vi "panelResize_tdms.vi"(4 "error in (no error)":errorcluster, 5 "NewBnds":T2, 7 "control refs":T1) -> (0 "error out":errorcluster)   [LabVIEW 2020]
uses:
  <vilib>/Utility/miscctls.llb/LVRectTypeDef.ctl
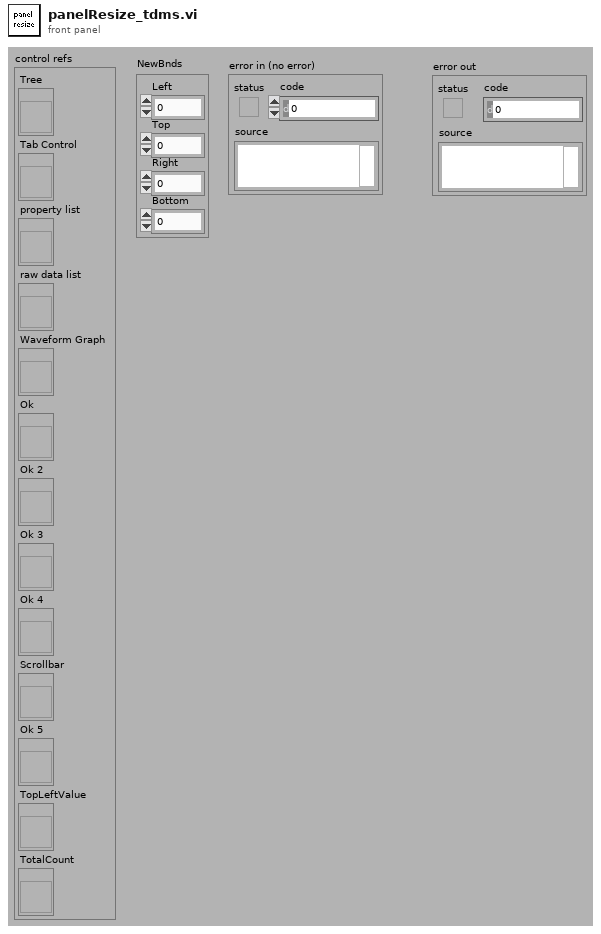
[diagram p1: front panel]
types:
  T1 = cluster{"Tree":refnum<vi>, "Tab Control":refnum<vi>, "property list":refnum<vi>, "raw data list":refnum<vi>, "Waveform Graph":refnum<vi>, "Ok":refnum<vi>, "Ok 2":refnum<vi>, "Ok 3":refnum<vi>, "Ok 4":refnum<vi>, "Scrollbar":refnum<vi>, "Ok 5":refnum<vi>, "TopLeftValue":refnum<vi>, "TotalCount":refnum<vi>}
  T2 = typedef "LVRectTypeDef.ctl" = cluster{"Left":i16, "Top":i16, "Right":i16, "Bottom":i16}
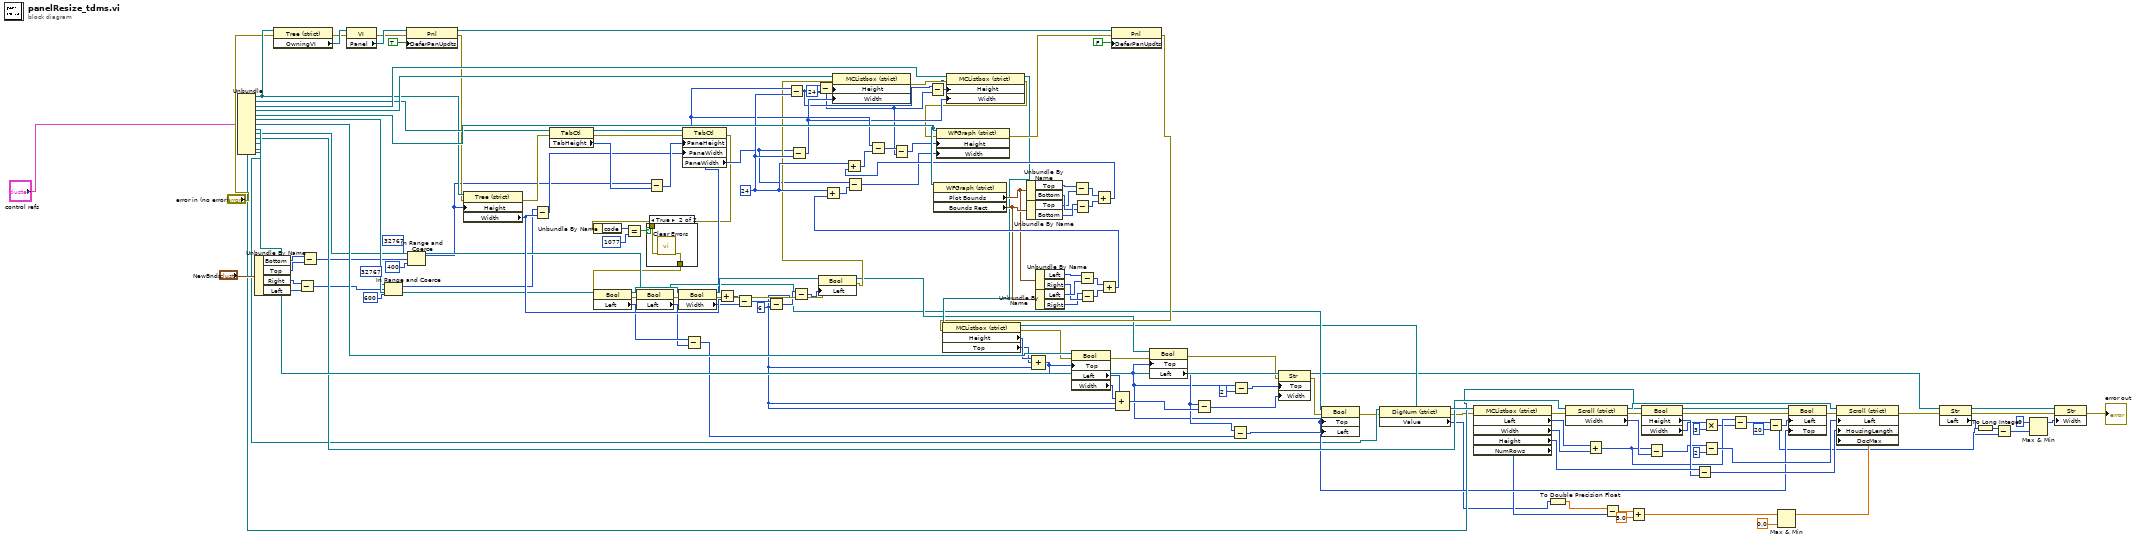
[diagram p0: block diagram]
diagram:
  w96 = u32 24 ("y")
  w77 = u32 6 ("y")
  w145 = u32 24 ("y")
  n1 = Unbundle("control refs") -> ("Tree"=w116:refnum<vi>, "Tab Control"=w152:refnum<vi>, "property list"=w153:refnum<vi>, "raw data list"=w154:refnum<vi>, "Waveform Graph"=w155:refnum<vi>, "Ok"=w76:refnum<vi>, "Ok 2"=w104:refnum<vi>, "Ok 3"=w87:refnum<vi>, "Ok 4"=w74:refnum<vi>, "Scrollbar"=w54:refnum<vi>, "Ok 5"=w50:refnum<vi>, "TotalCount"=w20:refnum<vi>)  [unwired: 1 out]
  n2 = Unbundle By Name("NewBnds") -> ("Bottom"=w123:i16, "Top"=w122:i16, "Right"=w150:i16, "Left"=w148:i16)
  n3 = property class="Tree (strict)"(reference=w116, error in="error in (no error)") -> (error out=w113:errorcluster, "OwningVI"=w115:refnum<vi>)  [unwired: 1 out]
  n4 = Subtract(x=w150, y=w148) -> (x-y=w24:i16)
  n5 = Subtract(x=w123, y=w122) -> (x-y=w30:i16)
  n6 = property class="VI"(reference=w115, error in=w113) -> (error out=w112:errorcluster, "Panel"=w114:refnum<vi>)  [unwired: 1 out]
  n7 = In Range and Coerce(upper limit=i16 32767, x=w24, lower limit=i16 600 ("upper limit")) -> (coerced(x)=w23:i16)  [unwired: 1 out]
  n8 = property class="Pnl"(reference=w114, error in=w112, "DeferPanUpdts"=TRUE ("Defer Panel Updates")) -> (reference out=w108:refnum<vi>, error out=w106:errorcluster)
  n9 = In Range and Coerce(upper limit=i16 32767, x=w30, lower limit=i16 400 ("upper limit")) -> (coerced(x)=w29:i16)  [unwired: 1 out]
  n10 = property class="Tree (strict)"(reference=w116, error in=w106, "Height"=w29) -> (error out=w119:errorcluster, "Width"=w105:u32)  [unwired: 1 out]
  n11 = Subtract(x=w23, y=w105) -> (x-y=w63:u32)
  n12 = property class="TabCtl"(reference=w152, error in=w119) -> (reference out=w124:refnum<vi>, error out=w62:errorcluster, "TabHeight"=w125:u32)
  n13 = Subtract(x=w29, y=w125) -> (x-y=w128:u32)
  n14 = property class="TabCtl"(reference=w124, error in=w62, "PaneHeight"=w128, "PaneWidth"=w63) -> (error out=w58:errorcluster, "PaneWidth"=w64:u32)  [unwired: 1 out]
  n15 = Unbundle By Name(w58) -> ("code"=w61:i32)
  n16 = Equal?(x=w61, y=1077) -> (x = y?=w59:bool)
  n17 = case shown="True" w59 {
    tunnel: w58 -> [w156 w158]
    tunnel: [w156 w157] -> w57
    frame False {
    }
    frame True {
      n18 = call <vilib>:"Clear Errors.vi"("error in (no error)"=w158) -> ("error out"=w157:errorcluster)  [unwired: 5 in, 1 out]
    }
  }
  n19 = property class="Bool"(reference=w76, error in=w57) -> (reference out=w75:refnum<vi>, error out=w73:errorcluster, "Left"=w68:i32)
  n20 = property class="Bool"(reference=w74, error in=w73) -> (reference out=w71:refnum<vi>, error out=w72:errorcluster, "Left"=w67:i32)
  n21 = property class="Bool"(reference=w75, error in=w72) -> (reference out=w149:refnum<vi>, error out=w120:errorcluster, "Width"=w102:u32)
  n22 = Subtract(x=w68, y=w67) -> (x-y=w66:i32)
  n23 = Add(x=w64, y=w105) -> (x+y=w103:u32)
  n24 = Subtract(x=w103, y=w102) -> (x-y=w151:u32)
  n25 = Subtract(x=w151, y=w77) -> (x-y=w79:u32)
  n26 = Subtract(x=w128, y=w145) -> (x-y=w97:u32)
  n27 = Subtract(x=w64, y=w145) -> (x-y=w126:u32)
  n28 = Subtract(x=w79, y=w77) -> (x-y=w78:u32)
  n29 = Subtract(x=w97, y=w96) -> (x-y=w99:u32)
  n30 = property class="Bool"(reference=w149, error in=w120, "Left"=w78) -> (reference out=w88:refnum<vi>, error out=w95:errorcluster)
  n31 = property class="MCListbox (strict)"(reference=w154, error in=w95, "Height"=w99, "Width"=w126) -> (error out=w118:errorcluster)  [unwired: 1 out]
  n32 = Subtract(x=w97, y=w96) -> (x-y=w98:u32)
  n33 = property class="WFGraph (strict)"(reference=w155) -> ("Plot Bounds"=w141:T2, "Bounds Rect"=w142:T2)  [unwired: 1 in, 2 out]
  n34 = property class="MCListbox (strict)"(reference=w153, error in=w118, "Height"=w98, "Width"=w126) -> (reference out=w94:refnum<vi>, error out=w117:errorcluster)
  n35 = Unbundle By Name(w141) -> ("Top"=w130:i16, "Bottom"=w131:i16)
  n36 = Unbundle By Name(w142) -> ("Top"=w129:i16, "Bottom"=w132:i16)
  n37 = Unbundle By Name(w141) -> ("Left"=w139:i16, "Right"=w138:i16)
  n38 = Unbundle By Name(w142) -> ("Left"=w140:i16, "Right"=w137:i16)
  n39 = Subtract(x=w130, y=w129) -> (x-y=w133:i16)
  n40 = Subtract(x=w132, y=w131) -> (x-y=w134:i16)
  n41 = Subtract(x=w139, y=w140) -> (x-y=w136:i16)
  n42 = Subtract(x=w137, y=w138) -> (x-y=w135:i16)
  n43 = Add(x=w133, y=w134) -> (x+y=w146:i16)
  n44 = Add(x=w145, y=w146) -> (x+y=w147:u32)
  n45 = Subtract(x=w128, y=w147) -> (x-y=w101:u32)
  n46 = Subtract(x=w101, y=w96) -> (x-y=w100:u32)
  n47 = Add(x=w136, y=w135) -> (x+y=w143:i16)
  n48 = Add(x=w145, y=w143) -> (x+y=w144:u32)
  n49 = Subtract(x=w64, y=w144) -> (x-y=w127:u32)
  n50 = property class="WFGraph (strict)"(reference=w155, error in=w117, "Height"=w100, "Width"=w127) -> (error out=w107:errorcluster)  [unwired: 1 out]
  n51 = property class="Pnl"(reference=w108, error in=w107, "DeferPanUpdts"=FALSE ("Defer Panel Updates")) -> (error out=w92:errorcluster)  [unwired: 1 out]
  n52 = property class="MCListbox (strict)"(reference=w94, error in=w92) -> (reference out=w55:refnum<vi>, error out=w93:errorcluster, "Height"=w91:u32, "Top"=w90:i32)
  n53 = Compound Arithmetic op=ADD(w91, w90, w77) -> (w31:u32)
  n54 = property class="Bool"(reference=w104, error in=w93, "Top"=w31) -> (error out=w89:errorcluster, "Left"=w84:i32, "Width"=w85:u32)  [unwired: 1 out]
  n55 = Compound Arithmetic op=ADD(w84, w85, w77, w77) -> (w83:u32)
  n56 = property class="Bool"(reference=w88, error in=w89, "Top"=w31) -> (error out=w86:errorcluster, "Left"=w69:i32)  [unwired: 1 out]
  n57 = Subtract(x=w69, y=w83) -> (x-y=w82:u32)
  n58 = Subtract(x=w69, y=w66) -> (x-y=w65:i32)
  n59 = Subtract(x=w31, y=u32 2) -> (x-y=w81:u32)
  n60 = property class="Str"(reference=w87, error in=w86, "Top"=w81, "Width"=w82) -> (reference out=w11:refnum<vi>, error out=w70:errorcluster)
  n61 = property class="Bool"(reference=w71, error in=w70, "Top"=w31, "Left"=w65) -> (error out=w19:errorcluster)  [unwired: 1 out]
  n62 = property class="DigNum (strict)"(reference=w20, error in=w19) -> (error out=w18:errorcluster, "Value"=w14:u64)  [unwired: 1 out]
  n63 = property class="MCListbox (strict)"(reference=w55, error in=w18) -> (error out=w44:errorcluster, "Left"=w52:i32, "Width"=w51:u32, "Height"=w49:u32, "NumRows"=w17:u32)  [unwired: 1 out]
  n64 = To Double Precision Float(number=w14) -> (double precision float=w13:dbl)
  n65 = property on="Property Node" class="Scroll (strict)"(reference=w54, error in=w44) -> (reference out=w53:refnum<vi>, error out=w43:errorcluster, "Width"=w46:u32)
  n66 = Add(x=w52, y=w51) -> (x+y=w37:u32)
  n67 = Subtract(x=w13, y=w17) -> (x-y=w22:dbl)
  n68 = Add(x=w22, y=5.0) -> (x+y=w16:dbl)
  n69 = property class="Bool"(reference=w50, error in=w43) -> (reference out=w47:refnum<vi>, error out=w42:errorcluster, "Height"=w48:u32, "Width"=w35:u32)
  n70 = Subtract(x=w37, y=w46) -> (x-y=w40:u32)
  n71 = Subtract(x=w49, y=w48) -> (x-y=w45:u32)
  n72 = Multiply(x=w35, y=u32 3) -> (x*y=w36:u32)
  n73 = Subtract(x=w40, y=u32 2) -> (x-y=w39:u32)
  n74 = Subtract(x=w37, y=w36) -> (x-y=w33:u32)
  n75 = Subtract(x=w33, y=u32 20) -> (x-y=w7:u32)
  n76 = Max & Min(x=w16, y=0.0) -> (max(x,y)=w15:dbl)  [unwired: 1 out]
  n77 = property class="Bool"(reference=w47, error in=w42, "Left"=w7, "Top"=w31) -> (error out=w41:errorcluster)  [unwired: 1 out]
  n78 = property on="Property Node" class="Scroll (strict)"(reference=w53, error in=w41, "Left"=w39, "HousingLength"=w45, "DocMax"=w15) -> (error out=w10:errorcluster)  [unwired: 1 out]
  n79 = property class="Str"(reference=w11, error in=w10) -> (reference out=w8:refnum<vi>, error out=w9:errorcluster, "Left"=w1:i32)
  n80 = To Long Integer(number=w7) -> (32bit integer=w2:i32)
  n81 = Subtract(x=w2, y=w1) -> (x-y=w6:i32)
  n82 = Max & Min(x=0, y=w6) -> (max(x,y)=w4:i32)  [unwired: 1 out]
  n83 = property class="Str"(reference=w8, error in=w9, "Width"=w4) -> (error out=→"error out":errorcluster)  [unwired: 1 out]
